vi "rsscope_core_global.vi"() -> ()   [LabVIEW 2014] (continued)
"Instrument Options"="", "Flags"=0, "Help"="Sets the duration of a line, the time between two successive sync pulses.\n\nAvailable Repeated Capabilities:\nNone\n\nRemote-control command(s):\nTRIGger<m>:TV:CUSTom:LDURation"}, {"Level"=3, "Class Only"=FALSE, "Identifier"="RSSCOPE_ATTR_TV_TRIGGER_PULSE_WIDTH", "Descriptive Name"="TV Trigger Pulse Width", "Data Type"=1, "Command"="TRIGger1:TV:CUST:SDUR", "Access"=2, "Range Table"="rsscope_rngTVPulseWidth", "Read Callback"="", "Write Callback"="", "Supported Models"="", "Instrument Options"="", "Flags"=0, "Help"="Sets the width of the sync pulse.\n\nAvailable Repeated Capabilities:\nNone\n\nRemote-control command(s):\nTRIGger<m>:TV:CUSTom:SDURation"}, {"Level"=3, "Class Only"=FALSE, "Identifier"="RSSCOPE_ATTR_TV_TRIGGER_SCAN_MODE", "Descriptive Name"="TV Trigger Scan Mode", "Data Type"=0, "Command"="TRIGger1:TV:CUST:SCAN", "Access"=2, "Range Table"="rsscope_rngTVScanMode", "Read Callback"="", "Write Callback"="", "Supported Models"="", "Instrument Options"="", "Flags"=0, "Help"="Sets the scanning system.\n\nAvailable Repeated Capabilities:\nNone\n\nRemote-control command(s):\nTRIGger<m>:TV:CUSTom:SCANmode"}, {"Level"=2, "Class Only"=TRUE, "Identifier"="", "Descriptive Name"="Trigger Qualification", "Data Type"=0, "Command"="", "Access"=0, "Range Table"="", "Read Callback"="", "Write Callback"="", "Supported Models"="", "Instrument Options"="", "Flags"=0, "Help"="By qualifying a trigger event, you can logically combine the trigger signal with the state of other digital channel signals.\nThe instrument triggers if both of the following apply:\n- The basic conditions of the trigger event definition are fulfilled.\n- The logical conditions of the trigger qualification are true.\n\nQualification is not supported with slew rate, Data2Clock, and serial pattern trigger types.\n\nThe A-event and B-event in a trigger sequence can have their own trigger qualification. Qualification is not available for R-events (Suffix m = 3).\n\nExample: Trigger on write access of a specific device of a bus system In circuits using SPI, several slave devices use the same lines for reading and writing data, and each slave has its own select line. To trigger on write access of specific slave, the write line is the trigger source and the select line of the slave is set as qualifiying."}, {"Level"=3, "Class Only"=FALSE, "Identifier"="RSSCOPE_ATTR_TRIGGER_QUALIFICATION_ENABLED", "Descriptive Name"="Trigger Qualification Enabled", "Data Type"=3, "Command"="TRIG{Trigger}:QUAL{TriggerType}:STAT", "Access"=2, "Range Table"="", "Read Callback"="", "Write Callback"="", "Supported Models"="", "Instrument Options"="", "Flags"=0, "Help"="Enables the use of the qualification definition for the selected trigger event.\n\nAvailable Repeated Capabilities:\nTrigger: TrigA, TrigB, TrigR\r\nTriggerType: Edge, Width, Runt, Glitch, Window, Timeout, Interval, Slew, Data2Clock, Pattern, External, T11, T12, NFC, TV, CDR\r\n\nRemote-control command(s):\nTRIGger<m>:QUALify<n>:STATe"}, {"Level"=3, "Class Only"=FALSE, "Identifier"="RSSCOPE_ATTR_TRIGGER_QUALIFICATION_ENABLED_CHANNEL_1", "Descriptive Name"="Trigger Qualification Enabled Channel 1", "Data Type"=3, "Command"="TRIG{Trigger}:QUAL{TriggerType}:A", "Access"=2, "Range Table"="", "Read Callback"="", "Write Callback"="", "Supported Models"="", "Instrument Options"="", "Flags"=0, "Help"="The command is relevant for qualification, for pattern trigger and for state trigger. The trigger source cannot be enabled.\n\nAvailable Repeated Capabilities:\nTrigger: TrigA, TrigB, TrigR\r\nTriggerType: Edge, Width, Runt, Glitch, Window, Timeout, Interval, Slew, Data2Clock, Pattern, External, T11, T12, NFC, TV, CDR\r\n\nRemote-control command(s):\nTRIGger<m>:QUALify<n>:A[:ENABle]"}, {"Level"=3, "Class Only"=FALSE, "Identifier"="RSSCOPE_ATTR_TRIGGER_QUALIFICATION_ENABLED_CHANNEL_2", "Descriptive Name"="Trigger Qualification Enabled Channel 2", "Data Type"=3, "Command"="TRIG{Trigger}:QUAL{TriggerType}:B", "Access"=2, "Range Table"="", "Read Callback"="", "Write Callback"="", "Supported Models"="", "Instrument Options"="", "Flags"=0, "Help"="The command is relevant for qualification, for pattern trigger and for state trigger. The trigger source cannot be enabled.\n\nAvailable Repeated Capabilities:\nTrigger: TrigA, TrigB, TrigR\r\nTriggerType: Edge, Width, Runt, Glitch, Window, Timeout, Interval, Slew, Data2Clock, Pattern, External, T11, T12, NFC, TV, CDR\r\n\nRemote-control command(s):\nTRIGger<m>:QUALify<n>:B[:ENABle]"}, {"Level"=3, "Class Only"=FALSE, "Identifier"="RSSCOPE_ATTR_TRIGGER_QUALIFICATION_ENABLED_CHANNEL_3", "Descriptive Name"="Trigger Qualification Enabled Channel 3", "Data Type"=3, "Command"="TRIG{Trigger}:QUAL{TriggerType}:C", "Access"=2, "Range Table"="", "Read Callback"="", "Write Callback"="", "Supported Models"="", "Instrument Options"="", "Flags"=0, "Help"="The command is relevant for qualification, for pattern trigger and for state trigger. The trigger source cannot be enabled.\n\nAvailable Repeated Capabilities:\nTrigger: TrigA, TrigB, TrigR\r\nTriggerType: Edge, Width, Runt, Glitch, Window, Timeout, Interval, Slew, Data2Clock, Pattern, External, T11, T12, NFC, TV, CDR\r\n\nRemote-control command(s):\nTRIGger<m>:QUALify<n>:C[:ENABle]"}, {"Level"=3, "Class Only"=FALSE, "Identifier"="RSSCOPE_ATTR_TRIGGER_QUALIFICATION_ENABLED_CHANNEL_4", "Descriptive Name"="Trigger Qualification Enabled Channel 4", "Data Type"=3, "Command"="TRIG{Trigger}:QUAL{TriggerType}:D", "Access"=2, "Range Table"="", "Read Callback"="", "Write Callback"="", "Supported Models"="", "Instrument Options"="", "Flags"=0, "Help"="The command is relevant for qualification, for pattern trigger and for state trigger. The trigger source cannot be enabled.\n\nAvailable Repeated Capabilities:\nTrigger: TrigA, TrigB, TrigR\r\nTriggerType: Edge, Width, Runt, Glitch, Window, Timeout, Interval, Slew, Data2Clock, Pattern, External, T11, T12, NFC, TV, CDR\r\n\nRemote-control command(s):\nTRIGger<m>:QUALify<n>:D[:ENABle]"}, {"Level"=3, "Class Only"=FALSE, "Identifier"="RSSCOPE_ATTR_TRIGGER_QUALIFICATION_LOGIC_CHANNEL_1", "Descriptive Name"="Trigger Qualification Logic Channel 1", "Data Type"=0, "Command"="TRIG{Trigger}:QUAL{TriggerType}:A:LOG", "Access"=2, "Range Table"="rsscope_rngTriggerQualificationLogic", "Read Callback"="", "Write Callback"="", "Supported Models"="", "Instrument Options"="", "Flags"=0, "Help"="Defines the logic for the indicated channel.\n\nAvailable Repeated Capabilities:\nTrigger: TrigA, TrigB, TrigR\r\nTriggerType: Edge, Width, Runt, Glitch, Window, Timeout, Interval, Slew, Data2Clock, Pattern, External, T11, T12, NFC, TV, CDR\r\n\nRemote-control command(s):\nTRIGger<m>:QUALify<n>:A:LOGic"}, {"Level"=3, "Class Only"=FALSE, "Identifier"="RSSCOPE_ATTR_TRIGGER_QUALIFICATION_LOGIC_CHANNEL_2", "Descriptive Name"="Trigger Qualification Logic Channel 2", "Data Type"=0, "Command"="TRIG{Trigger}:QUAL{TriggerType}:B:LOG", "Access"=2, "Range Table"="rsscope_rngTriggerQualificationLogic", "Read Callback"="", "Write Callback"="", "Supported Models"="", "Instrument Options"="", "Flags"=0, "Help"="Defines the logic for the indicated channel.\n\nAvailable Repeated Capabilities:\nTrigger: TrigA, TrigB, TrigR\r\nTriggerType: Edge, Width, Runt, Glitch, Window, Timeout, Interval, Slew, Data2Clock, Pattern, External, T11, T12, NFC, TV, CDR\r\n\nRemote-control command(s):\nTRIGger<m>:QUALify<n>:B:LOGic"}, {"Level"=3, "Class Only"=FALSE, "Identifier"="RSSCOPE_ATTR_TRIGGER_QUALIFICATION_LOGIC_CHANNEL_3", "Descriptive Name"="Trigger Qualification Logic Channel 3", "Data Type"=0, "Command"="TRIG{Trigger}:QUAL{TriggerType}:C:LOG", "Access"=2, "Range Table"="rsscope_rngTriggerQualificationLogic", "Read Callback"="", "Write Callback"="", "Supported Models"="", "Instrument Options"="", "Flags"=0, "Help"="Defines the logic for the indicated channel.\n\nAvailable Repeated Capabilities:\nTrigger: TrigA, TrigB, TrigR\r\nTriggerType: Edge, Width, Runt, Glitch, Window, Timeout, Interval, Slew, Data2Clock, Pattern, External, T11, T12, NFC, TV, CDR\r\n\nRemote-control command(s):\nTRIGger<m>:QUALify<n>:C:LOGic"}, {"Level"=3, "Class Only"=FALSE, "Identifier"="RSSCOPE_ATTR_TRIGGER_QUALIFICATION_LOGIC_CHANNEL_4", "Descriptive Name"="Trigger Qualification Logic Channel 4", "Data Type"=0, "Command"="TRIG{Trigger}:QUAL{TriggerType}:D:LOG", "Access"=2, "Range Table"="rsscope_rngTriggerQualificationLogic", "Read Callback"="", "Write Callback"="", "Supported Models"="", "Instrument Options"="", "Flags"=0, "Help"="Defines the logic for the indicated channel.\n\nAvailable Repeated Capabilities:\nTrigger: TrigA, TrigB, TrigR\r\nTriggerType: Edge, Width, Runt, Glitch, Window, Timeout, Interval, Slew, Data2Clock, Pattern, External, T11, T12, NFC, TV, CDR\r\n\nRemote-control command(s):\nTRIGger<m>:QUALify<n>:D:LOGic"}, {"Level"=3, "Class Only"=FALSE, "Identifier"="RSSCOPE_ATTR_TRIGGER_QUALIFICATION_LOGIC_CHANNELS_1_2", "Descriptive Name"="Trigger Qualification Logic Channels 1 2", "Data Type"=0, "Command"="TRIG{Trigger}:QUAL{TriggerType}:AB:LOG", "Access"=2, "Range Table"="rsscope_rngLogic", "Read Callback"="", "Write Callback"="", "Supported Models"="", "Instrument Options"="", "Flags"=0, "Help"="Defines the logical combination of the indicated channels after evaluating the previous logical operations.\n\nAvailable Repeated Capabilities:\nTrigger: TrigA, TrigB, TrigR\r\nTriggerType: Edge, Width, Runt, Glitch, Window, Timeout, Interval, Slew, Data2Clock, Pattern, External, T11, T12, NFC, TV, CDR\r\n\nRemote-control command(s):\nTRIGger<m>:QUALify<n>:AB:LOGic"}, {"Level"=3, "Class Only"=FALSE, "Identifier"="RSSCOPE_ATTR_TRIGGER_QUALIFICATION_LOGIC_CHANNELS_3_4", "Descriptive Name"="Trigger Qualification Logic Channels 3 4", "Data Type"=0, "Command"="TRIG{Trigger}:QUAL{TriggerType}:CD:LOG", "Access"=2, "Range Table"="rsscope_rngLogic", "Read Callback"="", "Write Callback"="", "Supported Models"="", "Instrument Options"="", "Flags"=0, "Help"="Defines the logical combination of the indicated channels after evaluating the previous logical operations.\n\nAvailable Repeated Capabilities:\nTrigger: TrigA, TrigB, TrigR\r\nTriggerType: Edge, Width, Runt, Glitch, Window, Timeout, Interval, Slew, Data2Clock, Pattern, External, T11, T12, NFC, TV, CDR\r\n\nRemote-control command(s):\nTRIGger<m>:QUALify<n>:CD:LOGic"}, {"Level"=3, "Class Only"=FALSE, "Identifier"="RSSCOPE_ATTR_TRIGGER_QUALIFICATION_LOGIC_CHANNELS_ALL", "Descriptive Name"="Trigger Qualification Logic Channels All", "Data Type"=0, "Command"="TRIG{Trigger}:QUAL{TriggerType}:ABCD:LOG", "Access"=2, "Range Table"="rsscope_rngLogic", "Read Callback"="", "Write Callback"="", "Supported Models"="", "Instrument Options"="", "Flags"=0, "Help"="Defines the logical combination of the indicated channels after evaluating the result of channels 1+2 and 3+4.\n\nAvailable Repeated Capabilities:\nTrigger: TrigA, TrigB, TrigR\r\nTriggerType: Edge, Width, Runt, Glitch, Window, Timeout, Interval, Slew, Data2Clock, Pattern, External, T11, T12, NFC, TV, CDR\r\n\nRemote-control command(s):\nTRIGger<m>:QUALify<n>:ABCD:LOGic"}, {"Level"=2, "Class Only"=TRUE, "Identifier"="", "Descriptive Name"="Noise Reject", "Data Type"=0, "Command"="", "Access"=0, "Range Table"="", "Read Callback"="", "Write Callback"="", "Supported Models"="", "Instrument Options"="", "Flags"=0, "Help"="The rejection of noise by settting a hysteresis avoids unwanted trigger events caused by noise oscillation around the trigger level. You can select the hysteresis mode and value for each channel, or couple the trigger levels and set the same hysteresis for all channels."}, {"Level"=3, "Class Only"=FALSE, "Identifier"="RSSCOPE_ATTR_NOISE_REJECT_HYSTERESIS_MODE", "Descriptive Name"="Noise Reject Hysteresis Mode", "Data Type"=0, "Command"="TRIG{Trigger}:LEV{TriggerSource}:NOIS", "Access"=2, "Range Table"="rsscope_rngAutoManual", "Read Callback"="", "Write Callback"="", "Supported Models"="", "Instrument Options"="", "Flags"=0, "Help"="Selects how the hysteresis is set.\n\nAvailable Repeated Capabilities:\nTrigger: TrigA, TrigB, TrigR\r\nTriggerSource: TsCH1, TsCH2, TsCH3, TsCH4, TsExt, TsLine, TsZ1V1, TsZ1V2, TsZ1V3, TsZ1V4, TsZ1I1, TsZ1I2, TsZ1I3, TsZ1I4, TsZ2V1, TsZ2V2, TsZ2V3, TsZ2V4, TsZ2I1, TsZ2I2, TsZ2I3, TsZ2I4, TsDiff1, TsDiff2, TsCommon1, TsCommon2\r\n\nRemote-control command(s):\nTRIGger<m>:LEVel<n>:NOISe[:STATe]"}, {"Level"=3, "Class Only"=FALSE, "Identifier"="RSSCOPE_ATTR_NOISE_REJECT_HYSTERESIS", "Descriptive Name"="Noise Reject Hysteresis", "Data Type"=1, "Command"="TRIG{Trigger}:LEV{TriggerSource}:NOIS:ABS", "Access"=2, "Range Table"="", "Read Callback"="", "Write Callback"="", "Supported Models"="", "Instrument Options"="", "Flags"=0, "Help"="Defines a range in absolute values around the trigger level. If the signal jitters inside this range and crosses the trigger level thereby, no trigger event occurs.\n\nAvailable Repeated Capabilities:\nTrigger: TrigA, TrigB, TrigR\r\nTriggerSource: TsCH1, TsCH2, TsCH3, TsCH4, TsExt, TsLine, TsZ1V1, TsZ1V2, TsZ1V3, TsZ1V4, TsZ1I1, TsZ1I2, TsZ1I3, TsZ1I4, TsZ2V1, TsZ2V2, TsZ2V3, TsZ2V4, TsZ2I1, TsZ2I2, TsZ2I3, TsZ2I4, TsDiff1, TsDiff2, TsCommon1, TsCommon2\r\n\nRemote-control command(s):\nTRIGger<m>:LEVel<n>:NOISe:ABSolute"}, {"Level"=3, "Class Only"=FALSE, "Identifier"="RSSCOPE_ATTR_NOISE_REJECT_HYSTERESIS_RELATIVE", "Descriptive Name"="Noise Reject Hysteresis Relative", "Data Type"=1, "Command"="TRIG{Trigger}:LEV{TriggerSource}:NOIS:REL", "Access"=2, "Range Table"="RsScope_rngNoiseRejectHysteresisRelative", "Read Callback"="", "Write Callback"="", "Supported Models"="", "Instrument Options"="", "Flags"=0, "Help"="Defines a range in percent around the trigger level. If the signal jitters inside this range and crosses the trigger level thereby, no trigger event occurs.\n\nAvailable Repeated Capabilities:\nTrigger: TrigA, TrigB, TrigR\r\nTriggerSource: TsCH1, TsCH2, TsCH3, TsCH4, TsExt, TsLine, TsZ1V1, TsZ1V2, TsZ1V3, TsZ1V4, TsZ1I1, TsZ1I2, TsZ1I3, TsZ1I4, TsZ2V1, TsZ2V2, TsZ2V3, TsZ2V4, TsZ2I1, TsZ2I2, TsZ2I3, TsZ2I4, TsDiff1, TsDiff2, TsCommon1, TsCommon2\r\n\nRemote-control command(s):\nTRIGger<m>:LEVel<n>:NOISe:RELative"}, {"Level"=3, "Class Only"=FALSE, "Identifier"="RSSCOPE_ATTR_NOISE_REJECT_HYSTERESIS_SCALE_MODE", "Descriptive Name"="Noise Reject Hysteresis Scale Mode", "Data Type"=0, "Command"="TRIG{Trigger}:LEV{TriggerSource}:NOIS:MODE", "Access"=2, "Range Table"="rsscope_rngAbsRel", "Read Callback"="", "Write Callback"="", "Supported Models"="", "Instrument Options"="", "Flags"=0, "Help"="Selects how the hysteresis is set.\n\nAvailable Repeated Capabilities:\nTrigger: TrigA, TrigB, TrigR\r\nTriggerSource: TsCH1, TsCH2, TsCH3, TsCH4, TsExt, TsLine, TsZ1V1, TsZ1V2, TsZ1V3, TsZ1V4, TsZ1I1, TsZ1I2, TsZ1I3, TsZ1I4, TsZ2V1, TsZ2V2, TsZ2V3, TsZ2V4, TsZ2I1, TsZ2I2, TsZ2I3, TsZ2I4, TsDiff1, TsDiff2, TsCommon1, TsCommon2\r\n\nRemote-control command(s):\nTRIGger<m>:LEVel<n>:NOISe:MODE"}, {"Level"=3, "Class Only"=FALSE, "Identifier"="RSSCOPE_ATTR_NOISE_REJECT_HYSTERESIS_RANGE_IN_DIVISIONS", "Descriptive Name"="Noise Reject Hysteresis Range In Divisions", "Data Type"=1, "Command"="TRIG{Trigger}:LEV{TriggerSource}:NOIS:PERD", "Access"=2, "Range Table"="RsScope_rngNoiseRejectHysteresisRangeInDivisions", "Read Callback"="", "Write Callback"="", "Supported Models"="", "Instrument Options"="", "Flags"=0, "Help"="Defines a range in divisions around the trigger level. If the signal oscillates inside this range and crosses the trigger level thereby, no trigger event occurs.\n\nAvailable Repeated Capabilities:\nTrigger: TrigA, TrigB, TrigR\r\nTriggerSource: TsCH1, TsCH2, TsCH3, TsCH4, TsExt, TsLine, TsZ1V1, TsZ1V2, TsZ1V3, TsZ1V4, TsZ1I1, TsZ1I2, TsZ1I3, TsZ1I4, TsZ2V1, TsZ2V2, TsZ2V3, TsZ2V4, TsZ2I1, TsZ2I2, TsZ2I3, TsZ2I4, TsDiff1, TsDiff2, TsCommon1, TsCommon2\r\n\nRemote-control command(s):\nTRIGger<m>:LEVel<n>:NOISe:PERDivision"}, {"Level"=2, "Class Only"=TRUE, "Identifier"="", "Descriptive Name"="Trigger Sequence", "Data Type"=0, "Command"="", "Access"=0, "Range Table"="", "Read Callback"="", "Write Callback"="", "Supported Models"="", "Instrument Options"="", "Flags"=0, "Help"="A trigger sequence consists of at least one trigger event and additional conditions defining when the trigger occurs. The simple sequence &apos;A only&apos; contains an A-event and the holdoff setting as optional condition. The complex trigger sequence &apos;A ? B ? R&apos; consists of two events - A and B - and an optional reset condition. After the A-event conditions have been met, the B-event with independent conditions is enabled. A- and B-events are configured in the same way. Without any reset, the instrument waits until one or a specified number of B-events occurs that causes the trigger, and then the sequence starts again. If you expect, for example, an irregular B-trigger event, you can configure a reset condition to restart the sequence with the A-event. The reset condition can be a simple timeout, or a trigger event that is defined in the same way as the A- and B-trigger events.\nThe instrument checks the trigger settings for compatibility and disables settings that do not fit the previous settings in the sequence."}, {"Level"=3, "Class Only"=FALSE, "Identifier"="RSSCOPE_ATTR_TRIGGER_SEQUENCE_MODE", "Descriptive Name"="Trigger Sequence Mode", "Data Type"=0, "Command"="TRIG:SEQ:TYPE", "Access"=2, "Range Table"="rsscope_rngTriggerSequence", "Read Callback"="", "Write Callback"="", "Supported Models"="", "Instrument Options"="", "Flags"=0, "Help"="Selects the type of the sequence.\n\nAvailable Repeated Capabilities:\nNone\n\nRemote-control command(s):\nTRIGger<m>:SEQuence:TYPE"}, {"Level"=3, "Class Only"=FALSE, "Identifier"="RSSCOPE_ATTR_TRIGGER_SEQUENCE_HOLDOFF_MODE", "Descriptive Name"="Trigger Sequence Holdoff Mode", "Data Type"=0, "Command"="TRIG:HOLD:MODE", "Access"=2, "Range Table"="rsscope_rngHoldoffMode", "Read Callback"="", "Write Callback"="", "Supported Models"="", "Instrument Options"="", "Flags"=0, "Help"="Selects the method to define the holdoff condition. The trigger holdoff defines when the next trigger after the current will be recognized. Thus, it affects the next trigger to occur after the current one. Holdoff helps to obtain stable triggering when the oscilloscope is triggering on undesired events.\n\nAvailable Repeated Capabilities:\nNone\n\nRemote-control command(s):\nTRIGger<m>:HOLDoff:MODE"}, {"Level"=3, "Class Only"=FALSE, "Identifier"="RSSCOPE_ATTR_TRIGGER_SEQUENCE_HOLDOFF_TIME", "Descriptive Name"="Trigger Sequence Holdoff Time", "Data Type"=1, "Command"="TRIG:HOLD:TIME", "Access"=2, "Range Table"="rsscope_rngInterval", "Read Callback"="", "Write Callback"="", "Supported Models"="", "Instrument Options"="", "Flags"=0, "Help"="Defines the holdoff time period. The next trigger occurs only after this time has passed. The setting is relevant if the holdoff mode is set to TIME.\n\nAvailable Repeated Capabilities:\nNone\n\nRemote-control command(s):\nTRIGger<m>:HOLDoff:TIME"}, {"Level"=3, "Class Only"=FALSE, "Identifier"="RSSCOPE_ATTR_TRIGGER_SEQUENCE_HOLDOFF_EVENTS", "Descriptive Name"="Trigger Sequence Holdoff Events", "Data Type"=0, "Command"="TRIG:HOLD:EVEN", "Access"=2, "Range Table"="", "Read Callback"="", "Write Callback"="", "Supported Models"="", "Instrument Options"="", "Flags"=0, "Help"="Defines the number of triggers to be skipped. The next trigger only occurs when this number of events is reached. The setting is relevant if the holdoff mode is set to EVENts.\n\nAvailable Repeated Capabilities:\nNone\n\nRemote-control command(s):\nTRIGger<m>:HOLDoff:EVENts"}, {"Level"=3, "Class Only"=FALSE, "Identifier"="RSSCOPE_ATTR_TRIGGER_SEQUENCE_HOLDOFF_RANDOM_MINIMUM_TIME", "Descriptive Name"="Trigger Sequence Holdoff Random Minimum Time", "Data Type"=1, "Command"="TRIG:HOLD:MIN", "Access"=2, "Range Table"="rsscope_rngRandomTimeMin", "Read Callback"="", "Write Callback"="", "Supported Models"="", "Instrument Options"="", "Flags"=0, "Help"="Defines the lower limit for the random time holdoff. The setting is relevant if the holdoff mode is set to RANDom.\n\nAvailable Repeated Capabilities:\nNone\n\nRemote-control command(s):\nTRIGger<m>:HOLDoff:MIN"}, {"Level"=3, "Class Only"=FALSE, "Identifier"="RSSCOPE_ATTR_TRIGGER_SEQUENCE_HOLDOFF_RANDOM_MAXIMUM_TIME", "Descriptive Name"="Trigger Sequence Holdoff Random Maximum Time", "Data Type"=1, "Command"="TRIG:HOLD:MAX", "Access"=2, "Range Table"="rsscope_rngInterval", "Read Callback"="", "Write Callback"="", "Supported Models"="", "Instrument Options"="", "Flags"=0, "Help"="Defines the lower limit for the random time holdoff. The setting is relevant if the holdoff mode is set to RANDom.\n\nAvailable Repeated Capabilities:\nNone\n\nRemote-control command(s):\nTRIGger<m>:HOLDoff:MAX"}, {"Level"=3, "Class Only"=FALSE, "Identifier"="RSSCOPE_ATTR_TRIGGER_SEQUENCE_HOLDOFF_AUTO_TIME_RESULT", "Descriptive Name"="Trigger Sequence Holdoff Auto Time Result", "Data Type"=1, "Command"="TRIG:HOLD:AUT?", "Access"=0, "Range Table"="", "Read Callback"="", "Write Callback"="", "Supported Models"="", "Instrument Options"="", "Flags"=0, "Help"="Returns the resulting holdoff time if the holdoff mode is set to AUTO: Auto time = Auto time scaling * Horizontal scale.\n\nAvailable Repeated Capabilities:\nNone\n\nRemote-control command(s):\nTRIGger<m>:HOLDoff:AUTotime?"}, {"Level"=3, "Class Only"=FALSE, "Identifier"="RSSCOPE_ATTR_TRIGGER_SEQUENCE_HOLDOFF_AUTO_SCALE", "Descriptive Name"="Trigger Sequence Holdoff Auto Scale", "Data Type"=1, "Command"="TRIG:HOLD:SCAL", "Access"=2, "Range Table"="rsscope_rngHoldoffAutoScale", "Read Callback"="", "Write Callback"="", "Supported Models"="", "Instrument Options"="", "Flags"=0, "Help"="Sets the auto time scaling factor the horizontal scale is multipied with: Auto time = Auto time scaling * Horizontal scale. The setting is relevant if the holdoff mode is set to AUTO.\n\nAvailable Repeated Capabilities:\nNone\n\nRemote-control command(s):\nTRIGger<m>:HOLDoff:SCALing"}, {"Level"=3, "Class Only"=FALSE, "Identifier"="RSSCOPE_ATTR_TRIGGER_SEQUENCE_DELAY", "Descriptive Name"="Trigger Sequence Delay", "Data Type"=1, "Command"="TRIG:SEQ:DEL", "Access"=2, "Range Table"="rsscope_rngTriggerSequenceDelay", "Read Callback"="", "Write Callback"="", "Supported Models"="", "Instrument Options"="", "Flags"=0, "Help"="Sets the time the instrument waits after an A-event until it recognizes B-events.\n\nAvailable Repeated Capabilities:\nNone\n\nRemote-control command(s):\nTRIGger<m>:SEQuence:DELay"}, {"Level"=3, "Class Only"=FALSE, "Identifier"="RSSCOPE_ATTR_TRIGGER_SEQUENCE_B_EVENTS_COUNT", "Descriptive Name"="Trigger Sequence B-Events Count", "Data Type"=0, "Command"="TRIG:SEQ:COUN", "Access"=2, "Range Table"="", "Read Callback"="", "Write Callback"="", "Supported Models"="", "Instrument Options"="", "Flags"=0, "Help"="Sets the number of B-events to be fulfilled after an A-event. The last B-event causes the trigger.\n\nAvailable Repeated Capabilities:\nNone\n\nRemote-control command(s):\nTRIGger<m>:SEQuence:COUNt"}, {"Level"=3, "Class Only"=FALSE, "Identifier"="RSSCOPE_ATTR_TRIGGER_SEQUENCE_RESET_BY_TIMEOUT_ENABLED", "Descriptive Name"="Trigger Sequence Reset By Timeout Enabled", "Data Type"=3, "Command"="TRIG:SEQ:RES:TIM", "Access"=2, "Range Table"="", "Read Callback"="", "Write Callback"="", "Supported Models"="", "Instrument Options"="", "Flags"=0, "Help"="If set to ON, the instrument waits for the time defined using TRIGger<m>:SEQuence:RESet:TIMeout:TIME for the specified number of B-events. If no trigger occurs during that time, the sequence is restarted with the A-event.\n\nAvailable Repeated Capabilities:\nNone\n\nRemote-control command(s):\nTRIGger<m>:SEQuence:RESet:TIMeout[:ENABle]"}, {"Level"=3, "Class Only"=FALSE, "Identifier"="RSSCOPE_ATTR_TRIGGER_SEQUENCE_RESET_TIMEOUT", "Descriptive Name"="Trigger Sequence Reset Timeout", "Data Type"=1, "Command"="TRIG:SEQ:RES:TIM:TIME", "Access"=2, "Range Table"="rsscope_rngTriggerSequenceDelay", "Read Callback"="", "Write Callback"="", "Supported Models"="", "Instrument Options"="", "Flags"=0, "Help"="The time the instrument waits for the number of B-events specified using TRIGger<m>:SEQuence:COUNt before the sequence is restarted with the A-event.\n\nAvailable Repeated Capabilities:\nNone\n\nRemote-control command(s):\nTRIGger<m>:SEQuence:RESet:TIMeout:TIME"}, {"Level"=3, "Class Only"=FALSE, "Identifier"="RSSCOPE_ATTR_TRIGGER_SEQUENCE_RESET_EVENT_ENABLED", "Descriptive Name"="Trigger Sequence Reset Event Enabled", "Data Type"=3, "Command"="TRIG:SEQ:RES:EVEN", "Access"=2, "Range Table"="", "Read Callback"="", "Write Callback"="", "Supported Models"="", "Instrument Options"="", "Flags"=0, "Help"="If set to ON, the trigger sequence is restarted by the R-event if the specified number of B-event does not occur.\n\nAvailable Repeated Capabilities:\nNone\n\nRemote-control command(s):\nTRIGger<m>:SEQuence:RESet:EVENt"}, {"Level"=2, "Class Only"=TRUE, "Identifier"="", "Descriptive Name"="I2C", "Data Type"=0, "Command"="", "Access"=0, "Range Table"="", "Read Callback"="", "Write Callback"="", "Supported Models"="", "Instrument Options"="", "Flags"=0, "Help"="Configures I2C trigger settings."}, {"Level"=3, "Class Only"=FALSE, "Identifier"="RSSCOPE_ATTR_PROTOCOL_I2C_TRIGGER_MODE", "Descriptive Name"="Protocol I2C Trigger Mode", "Data Type"=0, "Command"="TRIG{Trigger}:I2C:MODE", "Access"=2, "Range Table"="rsscope_rngProtocolI2CTriggerType", "Read Callback"="", "Write Callback"="", "Supported Models"="", "Instrument Options"="", "Flags"=0, "Help"="Selects the trigger type for I2C analysis.\n\nAvailable Repeated Capabilities:\nTrigger: TrigA, TrigB, TrigR\r\n\nRemote-control command(s):\nTRIGger<m>:I2C:MODE"}, {"Level"=3, "Class Only"=FALSE, "Identifier"="RSSCOPE_ATTR_PROTOCOL_I2C_TRIGGER_ADDRESS_NACK", "Descriptive Name"="Protocol I2C Trigger Address Nack", "Data Type"=3, "Command"="TRIG{Trigger}:I2C:ADN", "Access"=2, "Range Table"="", "Read Callback"="", "Write Callback"="", "Supported Models"="", "Instrument Options"="", "Flags"=0, "Help"="Triggers if the address acknowledge bit is missing - no slave recognizes the address.\n\nAvailable Repeated Capabilities:\nTrigger: TrigA, TrigB, TrigR\r\n\nRemote-control command(s):\nTRIGger<m>:I2C:ADNack"}, {"Level"=3, "Class Only"=FALSE, "Identifier"="RSSCOPE_ATTR_PROTOCOL_I2C_TRIGGER_DATA_WRITE_NACK", "Descriptive Name"="Protocol I2C Trigger Data Write Nack", "Data Type"=3, "Command"="TRIG{Trigger}:I2C:DWN", "Access"=2, "Range Table"="", "Read Callback"="", "Write Callback"="", "Supported Models"="", "Instrument Options"="", "Flags"=0, "Help"="Triggers if a date acknowledge bit is missing - the addressed slave does not accept the data.\n\nAvailable Repeated Capabilities:\nTrigger: TrigA, TrigB, TrigR\r\n\nRemote-control command(s):\nTRIGger<m>:I2C:DWNack"}, {"Level"=3, "Class Only"=FALSE, "Identifier"="RSSCOPE_ATTR_PROTOCOL_I2C_TRIGGER_DATA_READ_NACK", "Descriptive Name"="Protocol I2C Trigger Data Read Nack", "Data Type"=3, "Command"="TRIG{Trigger}:I2C:DRN", "Access"=2, "Range Table"="", "Read Callback"="", "Write Callback"="", "Supported Models"="", "Instrument Options"="", "Flags"=0, "Help"="Triggers on the end of the read process when the master reads data from the slave. This Nack is sent according to the protocol definition, it is not an error.\n\nAvailable Repeated Capabilities:\nTrigger: TrigA, TrigB, TrigR\r\n\nRemote-control command(s):\nTRIGger<m>:I2C:DRNack"}, {"Level"=3, "Class Only"=FALSE, "Identifier"="RSSCOPE_ATTR_PROTOCOL_I2C_TRIGGER_ACCESS_BIT", "Descriptive Name"="Protocol I2C Trigger Access Bit", "Data Type"=0, "Command"="TRIG{Trigger}:I2C:ACC", "Access"=2, "Range Table"="rsscope_rngProtocolI2CAccessBit", "Read Callback"="", "Write Callback"="", "Supported Models"="", "Instrument Options"="", "Flags"=0, "Help"="Sets the trigger condition for the R/W bit - the transfer direction of the data.\n\nAvailable Repeated Capabilities:\nTrigger: TrigA, TrigB, TrigR\r\n\nRemote-control command(s):\nTRIGger<m>:I2C:ACCess"}, {"Level"=3, "Class Only"=FALSE, "Identifier"="RSSCOPE_ATTR_PROTOCOL_I2C_TRIGGER_ADDRESS_TYPE", "Descriptive Name"="Protocol I2C Trigger Address Type", "Data Type"=0, "Command"="TRIG{Trigger}:I2C:AMOD", "Access"=2, "Range Table"="rsscope_rngProtocolI2CAddressType", "Read Callback"="", "Write Callback"="", "Supported Models"="", "Instrument Options"="", "Flags"=0, "Help"="Triggers on the address length.\n\nAvailable Repeated Capabilities:\nTrigger: TrigA, TrigB, TrigR\r\n\nRemote-control command(s):\nTRIGger<m>:I2C:AMODe"}, {"Level"=3, "Class Only"=FALSE, "Identifier"="RSSCOPE_ATTR_PROTOCOL_I2C_TRIGGER_ADDRESS_CONDITION", "Descriptive Name"="Protocol I2C Trigger Address Condition", "Data Type"=0, "Command"="TRIG{Trigger}:I2C:ACON", "Access"=2, "Range Table"="rsscope_rngProtocolTriggerCondition", "Read Callback"="", "Write Callback"="", "Supported Models"="", "Instrument Options"="", "Flags"=0, "Help"="Sets the operator to set a specific address or an address range.\n\nAvailable Repeated Capabilities:\nTrigger: TrigA, TrigB, TrigR\r\n\nRemote-control command(s):\nTRIGger<m>:I2C:ACONdition"}, {"Level"=3, "Class Only"=FALSE, "Identifier"="RSSCOPE_ATTR_PROTOCOL_I2C_TRIGGER_ADDRESS_MIN", "Descriptive Name"="Protocol I2C Trigger Address Min", "Data Type"=2, "Command"="TRIG{Trigger}:I2C:ADDR", "Access"=2, "Range Table"="", "Read Callback"="", "Write Callback"="", "Supported Models"="", "Instrument Options"="", "Flags"=0, "Help"="Triggers on the specified slave address, or sets the start value of an address range.\n\nValid Values: \nBinary pattern string consisting 1; 0; or X (any bit).\n\nAvailable Repeated Capabilities:\nTrigger: TrigA, TrigB, TrigR\r\n\nRemote-control command(s):\nTRIGger<m>:I2C:ADDRess"}, {"Level"=3, "Class Only"=FALSE, "Identifier"="RSSCOPE_ATTR_PROTOCOL_I2C_TRIGGER_ADDRESS_MAX", "Descriptive Name"="Protocol I2C Trigger Address Max", "Data Type"=2, "Command"="TRIG{Trigger}:I2C:ADDT", "Access"=2, "Range Table"="", "Read Callback"="", "Write Callback"="", "Supported Models"="", "Instrument Options"="", "Flags"=0, "Help"="Sets the end value of an address range.\n\nValid Values: \nBinary pattern string consisting 1 and 0.\n\nAvailable Repeated Capabilities:\nTrigger: TrigA, TrigB, TrigR\r\n\nRemote-control command(s):\nTRIGger<m>:I2C:ADDTo"}, {"Level"=3, "Class Only"=FALSE, "Identifier"="RSSCOPE_ATTR_PROTOCOL_I2C_TRIGGER_POSITION_CONDITION", "Descriptive Name"="Protocol I2C Trigger Position Condition", "Data Type"=0, "Command"="TRIG{Trigger}:I2C:DPOP", "Access"=2, "Range Table"="rsscope_rngI2CPositionCondition", "Read Callback"="", "Write Callback"="", "Supported Models"="", "Instrument Options"="", "Flags"=0, "Help"="Sets the operator for the data position.\n\nAvailable Repeated Capabilities:\nTrigger: TrigA, TrigB, TrigR\r\n\nRemote-control command(s):\nTRIGger<m>:I2C:DPOPerator"}, {"Level"=3, "Class Only"=FALSE, "Identifier"="RSSCOPE_ATTR_PROTOCOL_I2C_TRIGGER_POSITION_MIN", "Descriptive Name"="Protocol I2C Trigger Position Min", "Data Type"=0, "Command"="TRIG{Trigger}:I2C:DPOS", "Access"=2, "Range Table"="rsscope_rnglI2CPositionMinMax", "Read Callback"="", "Write Callback"="", "Supported Models"="", "Instrument Options"="", "Flags"=0, "Help"="Sets the number of data bytes before the first byte of interest. These bytes are ignored.\n\nAvailable Repeated Capabilities:\nTrigger: TrigA, TrigB, TrigR\r\n\nRemote-control command(s):\nTRIGger<m>:I2C:DPOSition"}, {"Level"=3, "Class Only"=FALSE, "Identifier"="RSSCOPE_ATTR_PROTOCOL_I2C_TRIGGER_POSITION_MAX", "Descriptive Name"="Protocol I2C Trigger Position Max", "Data Type"=0, "Command"="TRIG{Trigger}:I2C:DPTO", "Access"=2, "Range Table"="rsscope_rnglI2CPositionMinMax", "Read Callback"="", "Write Callback"="", "Supported Models"="", "Instrument Options"="", "Flags"=0, "Help"="Defines the last byte of interest.\n\nAvailable Repeated Capabilities:\nTrigger: TrigA, TrigB, TrigR\r\n\nRemote-control command(s):\nTRIGger<m>:I2C:DPTO"}, {"Level"=3, "Class Only"=FALSE, "Identifier"="RSSCOPE_ATTR_PROTOCOL_I2C_TRIGGER_DATA_CONDITION", "Descriptive Name"="Protocol I2C Trigger Data Condition", "Data Type"=0, "Command"="TRIG{Trigger}:I2C:DCON", "Access"=2, "Range Table"="rsscope_rngProtocolTriggerCondition", "Read Callback"="", "Write Callback"="", "Supported Models"="", "Instrument Options"="", "Flags"=0, "Help"="Sets the operator to set a specific address or an address range.\n\nAvailable Repeated Capabilities:\nTrigger: TrigA, TrigB, TrigR\r\n\nRemote-control command(s):\nTRIGger<m>:I2C:DCONdition"}, {"Level"=3, "Class Only"=FALSE, "Identifier"="RSSCOPE_ATTR_PROTOCOL_I2C_TRIGGER_PATTERN_MIN", "Descriptive Name"="Protocol I2C Trigger Pattern Min", "Data Type"=2, "Command"="TRIG{Trigger}:I2C:DMIN", "Access"=2, "Range Table"="", "Read Callback"="", "Write Callback"="", "Supported Models"="", "Instrument Options"="", "Flags"=0, "Help"="Specifies the data bit pattern, or sets the start value of a data pattern range.. Enter the bytes in msb first bit order. The maximum pattern length is 64 bit. Waveform data is compared with the pattern byte-by-byte.\n\nAvailable Repeated Capabilities:\nTrigger: TrigA, TrigB, TrigR\r\n\nRemote-control command(s):\nTRIGger<m>:I2C:DMIN"}, {"Level"=3, "Class Only"=FALSE, "Identifier"="RSSCOPE_ATTR_PROTOCOL_I2C_TRIGGER_PATTERN_MAX", "Descriptive Name"="Protocol I2C Trigger Pattern Max", "Data Type"=2, "Command"="TRIG{Trigger}:I2C:DMAX", "Access"=2, "Range Table"="", "Read Callback"="", "Write Callback"="", "Supported Models"="", "Instrument Options"="", "Flags"=0, "Help"="Sets the end value of an data range.\n\nAvailable Repeated Capabilities:\nTrigger: TrigA, TrigB, TrigR\r\n\nRemote-control command(s):\nTRIGger<m>:I2C:DMAX"}, {"Level"=3, "Class Only"=TRUE, "Identifier"="", "Descriptive Name"="OR Slot", "Data Type"=0, "Command"="", "Access"=0, "Range Table"="", "Read Callback"="", "Write Callback"="", "Supported Models"="", "Instrument Options"="", "Flags"=0, "Help"="Index of the address in an &apos;address OR&apos; condition (OR slot)"}, {"Level"=4, "Class Only"=FALSE, "Identifier"="RSSCOPE_ATTR_PROTOCOL_I2C_TRIGGER_ADDRESS_OR_STATE", "Descriptive Name"="Protocol I2C Trigger Address OR State", "Data Type"=3, "Command"="TRIG{Trigger}:I2C:ADOR{ORSlot}:ENAB", "Access"=2, "Range Table"="", "Read Callback"="", "Write Callback"="", "Supported Models"="", "Instrument Options"="", "Flags"=2, "Help"="This attribute sets the state of the selected address OR slot for the &apos;address OR&apos; trigger condition\n\nAvailable Repeated Capabilities:\nTrigger: TrigA, TrigB, TrigR\r\nORSlot: ORSlot1, ORSlot2, ORSlot3, ORSlot4\r\n\nRemote-control command(s):\nTRIGger<m>:I2C:ADOR<n>:ENABle"}, {"Level"=4, "Class Only"=FALSE, "Identifier"="RSSCOPE_ATTR_PROTOCOL_I2C_TRIGGER_ADDRESS_OR_TYPE", "Descriptive Name"="Protocol I2C Trigger Address OR Type", "Data Type"=0, "Command"="TRIG{Trigger}:I2C:ADOR{ORSlot}:ADRT", "Access"=2, "Range Table"="rsscope_rngProtocolI2CAddressORType", "Read Callback"="", "Write Callback"="", "Supported Models"="", "Instrument Options"="", "Flags"=0, "Help"="This attribute select address length.\n\nAvailable Repeated Capabilities:\nTrigger: TrigA, TrigB, TrigR\r\nORSlot: ORSlot1, ORSlot2, ORSlot3, ORSlot4\r\n\nRemote-control command(s):\nTRIGger<m>:I2C:ADOR<n>:ADRType"}, {"Level"=4, "Class Only"=FALSE, "Identifier"="RSSCOPE_ATTR_PROTOCOL_I2C_TRIGGER_ADDRESS_OR_ACCESS_BIT", "Descriptive Name"="Protocol I2C Trigger Address OR Access Bit", "Data Type"=0, "Command"="TRIG{Trigger}:I2C:ADOR{ORSlot}:RWB", "Access"=2, "Range Table"="rsscope_rngProtocolI2CAccessBit", "Read Callback"="", "Write Callback"="", "Supported Models"="", "Instrument Options"="", "Flags"=0, "Help"="Sets the R/W bit of the indicated ADOR address in the &apos;address OR&apos; trigger condition.\n\nAvailable Repeated Capabilities:\nTrigger: TrigA, TrigB, TrigR\r\nORSlot: ORSlot1, ORSlot2, ORSlot3, ORSlot4\r\n\nRemote-control command(s):\nTRIGger<m>:I2C:ADOR<n>:RWBit"}, {"Level"=4, "Class Only"=FALSE, "Identifier"="RSSCOPE_ATTR_PROTOCOL_I2C_TRIGGER_ADDRESS_OR", "Descriptive Name"="Protocol I2C Trigger Address OR", "Data Type"=2, "Command"="TRIG{Trigger}:I2C:ADOR{ORSlot}", "Access"=2, "Range Table"="", "Read Callback"="", "Write Callback"="", "Supported Models"="", "Instrument Options"="", "Flags"=0, "Help"="Setst the address pattern of the address.\n\nValid Values: \nBinary pattern string consisting 1; 0; or X (any bit).\n\nAvailable Repeated Capabilities:\nTrigger: TrigA, TrigB, TrigR\r\nORSlot: ORSlot1, ORSlot2, ORSlot3, ORSlot4\r\n\nRemote-control command(s):\nTRIGger<m>:I2C:ADOR<n>[:VALue]"}, {"Level"=2, "Class Only"=TRUE, "Identifier"="", "Descriptive Name"="SPI", "Data Type"=0, "Command"="", "Access"=0, "Range Table"="", "Read Callback"="", "Write Callback"="", "Supported Models"="", "Instrument Options"="", "Flags"=0, "Help"="Configures SPI trigger settings."}, {"Level"=3, "Class Only"=FALSE, "Identifier"="RSSCOPE_ATTR_PROTOCOL_SPI_TRIGGER_MODE", "Descriptive Name"="Protocol SPI Trigger Mode", "Data Type"=0, "Command"="TRIG:SPI:MODE", "Access"=2, "Range Table"="rsscope_rngProtocolSPITriggerType", "Read Callback"="", "Write Callback"="", "Supported Models"="", "Instrument Options"="", "Flags"=0, "Help"="Selects the trigger type for SPI analysis.\n\nAvailable Repeated Capabilities:\nNone\n\nRemote-control command(s):\nTRIGger<m>:SPI:MODE"}, {"Level"=3, "Class Only"=FALSE, "Identifier"="RSSCOPE_ATTR_PROTOCOL_SPI_TRIGGER_POSITION_CONDITION", "Descriptive Name"="Protocol SPI Trigger Position Condition", "Data Type"=0, "Command"="TRIG{Trigger}:SPI:DPOP", "Access"=2, "Range Table"="rsscope_rngSPIPositionCondition", "Read Callback"="", "Write Callback"="", "Supported Models"="", "Instrument Options"="", "Flags"=0, "Help"="Sets the operator for the data position. You can defined an exact position, or a position range.\n\nAvailable Repeated Capabilities:\nTrigger: TrigA, TrigB, TrigR\r\n\nRemote-control command(s):\nTRIGger<m>:SPI:DPOPerator"}, {"Level"=3, "Class Only"=FALSE, "Identifier"="RSSCOPE_ATTR_PROTOCOL_SPI_TRIGGER_DATA_ALIGNMENT", "Descriptive Name"="Protocol SPI Trigger Data Alignment", "Data Type"=0, "Command"="TRIG{Trigger}:SPI:PAL", "Access"=2, "Range Table"="rsscope_rngProtocolSPIDataAlignment", "Read Callback"="", "Write Callback"="", "Supported Models"="", "Instrument Options"="", "Flags"=0, "Help"="Defines how the specified data pattern is searched.\n\nAvailable Repeated Capabilities:\nTrigger: TrigA, TrigB, TrigR\r\n\nRemote-control command(s):\nTRIGger<m>:SPI:PALignment"}, {"Level"=3, "Class Only"=FALSE, "Identifier"="RSSCOPE_ATTR_PROTOCOL_SPI_TRIGGER_DATA_INDEX_MIN", "Descriptive Name"="Protocol SPI Trigger Data Index Min", "Data Type"=0, "Command"="TRIG{Trigger}:SPI:DPOS", "Access"=2, "Range Table"="rsscope_rngProtocolSPITriggerDataIndexMin", "Read Callback"="", "Write Callback"="", "Supported Models"="", "Instrument Options"="", "Flags"=0, "Help"="Sets the number of bits or words before the first word of interest.\n\nAvailable Repeated Capabilities:\nTrigger: TrigA, TrigB, TrigR\r\n\nRemote-control command(s):\nTRIGger<m>:SPI:DPOSition"}, {"Level"=3, "Class Only"=FALSE, "Identifier"="RSSCOPE_ATTR_PROTOCOL_SPI_TRIGGER_DATA_INDEX_MAX", "Descriptive Name"="Protocol SPI Trigger Data Index Max", "Data Type"=0, "Command"="TRIG{Trigger}:SPI:DPTO", "Access"=2, "Range Table"="rsscope_rngProtocolSPITriggerOffset", "Read Callback"="", "Write Callback"="", "Supported Models"="", "Instrument Options"="", "Flags"=0, "Help"="Defines the last byte of interest,if &apos;Condition&apos; is &apos;Range&apos;.\n\nAvailable Repeated Capabilities:\nTrigger: TrigA, TrigB, TrigR\r\n\nRemote-control command(s):\nTRIGger<m>:SPI:DPTO"}, {"Level"=3, "Class Only"=FALSE, "Identifier"="RSSCOPE_ATTR_PROTOCOL_SPI_TRIGGER_CONDITION", "Descriptive Name"="Protocol SPI Trigger Condition", "Data Type"=0, "Command"="TRIG{Trigger}:SPI:FCON", "Access"=2, 
